vi "Send Start.vi"(8 "error in (no error)":errorcluster, 11 "Plugin Interface in":refnum<class "Plugin Interface.lvclass">) -> (0 "error out":errorcluster, 3 "Plugin Interface out":refnum<class "Plugin Interface.lvclass">)   [LabVIEW 2021, in "DSF Core.lvlib" / "Plugin Interface.lvclass"]
uses:
  Plugin Interface.lvclass
  C:/dev/git/custom-devices/niveristand-data-sharing-framework-custom-device/Source/Core/Classes/Interface/Interface.lvclass
  Command.ctl
  Command Data.ctl
  Command Parameters.ctl
  Response.ctl
  Send Plugin Command.vi
  Wait For Plugin Response.vi
  Dispatcher/Invalid Response.vi
  Interface.lvclass
  DSF Core.lvlib
  C:/dev/git/custom-devices/niveristand-data-sharing-framework-custom-device/Source/Core/Classes/Interface/Plugin/Plugin Interface.lvclass
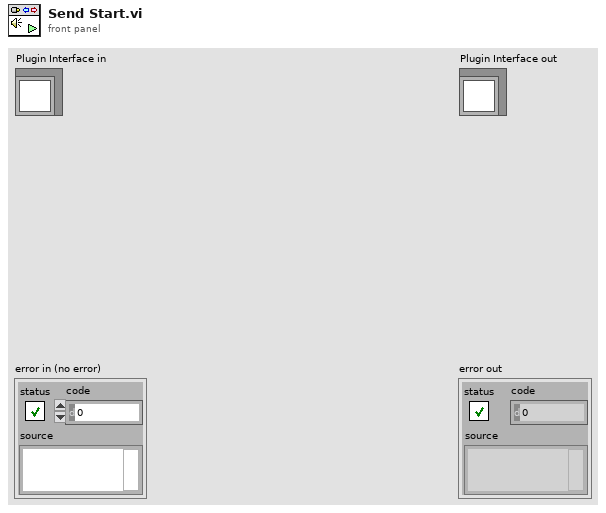
[diagram p1: front panel]
types:
  T1 = typedef "DSF Core.lvlib/Plugin Interface.lvclass/Command.ctl" = enum8{"Idle", "Start", "Set Inline Buffer", "Rx", "Tx", "Shutdown", "Error"}
  T2 = typedef "DSF Core.lvlib/Plugin Interface.lvclass/Command Data.ctl" = cluster{"Command":T1, "Parameters":T3}
  T3 = typedef "DSF Core.lvlib/Plugin Interface.lvclass/Command Parameters.ctl" = cluster{"arg1":u64, "arg2":u64}
  T4 = typedef "DSF Core.lvlib/Plugin Interface.lvclass/Response Data.ctl" = cluster{"Response":T5, "Parameters":T6}
  T5 = typedef "DSF Core.lvlib/Plugin Interface.lvclass/Response.ctl" = enum8{"General Ack", "Shutting Down"}
  T6 = typedef "DSF Core.lvlib/Plugin Interface.lvclass/Response Parameters.ctl" = cluster{"arg1":u64, "arg2":u64}
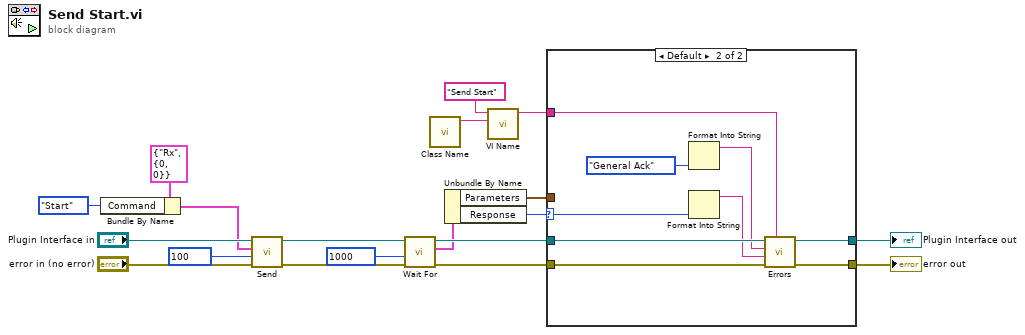
[diagram p0: block diagram]
diagram:
  n1 = Bundle By Name(cluster=T2 {"Command"=enum."Rx", "Parameters"={"arg1"=0, "arg2"=0}} ("command"), "Command"=Command."Start") -> (w15:T2)
  n2 = call-poly "Send.vi"("error in (no error)"="error in (no error)", "timeout in ms (0)"=100, "command"=w15, "Plugin Interface in"="Plugin Interface in") -> ("error out"=w13:errorcluster, "Plugin Interface out"=w14:refnum<class "Plugin Interface.lvclass">)  [unwired: 6 in]
  n3 = call-poly "Wait For.vi"("error in (no error)"=w13, "timeout in ms (0)"=1000, "Plugin Interface in"=w14) -> ("error out"=w9:errorcluster, "response"=w7:T4, "Plugin Interface out"=w11:refnum<class "Plugin Interface.lvclass">)  [unwired: 5 in, 1 out]
  n4 = call "Class Name.vi"() -> ("class name"=w3:string)  [unwired: 11 in]
  n5 = Unbundle By Name(w7) -> ("Parameters"=w5:T6, "Response"=w6:T5)
  n6 = call "VI Name.vi"("class name (\"\")"=w3, "vi name"="Send Start" ("error source vi name")) -> ("full VI name"=w1:string)  [unwired: 9 in]
  n7 = case shown="Default" w6 {
    selector: w6 -> [_ w26]
    tunnel: w11 -> [w21 w30]
    tunnel: [w21 w28] -> w10
    tunnel: w9 -> [w20 w29]
    tunnel: [w20 w27] -> w8
    tunnel: w5 -> [_ _]
    tunnel: w1 -> [_ w22]
    frame "General Ack" {
    }
    frame Default {
      n8 = Format Into String(Response."General Ack" ("Response")) -> (resulting string=w23:string)  [unwired: 3 in, 1 out]
      n9 = Format Into String(w26) -> (resulting string=w25:string)  [unwired: 3 in, 1 out]
      n10 = call-poly "Errors.vi"("error source vi name"=w22, "error in (no error)"=w29, "actual response"=w25, "expected response"=w23, "Interface in"=w30) -> ("error out"=w27:errorcluster, "Interface out"=w28:refnum<class "Plugin Interface.lvclass">)  [unwired: 5 in]
    }
  }
  "error out" <- w8
  "Plugin Interface out" <- w10
